vi "Send Initialize Parameters.vi"(7 "Message Priority (Normal)":T2=enum."Normal", 8 "error in (no error)":errorcluster, 10 "Cluster":T1={"Save Options"={"Primary Storage Location"=path "", "Backup Storage Location"=path "", "Enable Primary"=FALSE, "Enable Secondary"=FALSE, "Save Image as"=enum."RAW"}, "Other Settings"={"Show Image Averaging Option"=TRUE, "Component Name Prefix"=""}, "PLC Parameters"={"Initialize Parameters"={"VISA  Port"="", "Baud Rate"=0}, "Wakeup Bit (Set)"={"Address"=0, "Set/Reset"=FALSE}, "Incoming Bit (Get)"={"Address"=0, "Set/Reset"=FALSE}, "Acknowledge Bit (Set)"={"Address"=0, "Set/Reset"=FALSE}}}, 11 "Message Enqueuer":refnum<class "Message Enqueuer.lvclass">) -> (0 "error out":errorcluster, 3 "Message Enqueuer out":refnum<class "Message Enqueuer.lvclass">)   [LabVIEW 2022 SP3, in "Controller.lvlib" / "Initialize Parameters Msg.lvclass"]
doc: "This VI sends the message to an actor."
uses:
  Initialize Parameters Msg.lvclass
  <vilib>/ActorFramework/Message Enqueuer/Message Enqueuer.lvclass
  <vilib>/ActorFramework/Message Enqueuer/Message Priority.ctl
  C:/Program Files/National Instruments/LabVIEW 2022/vi.lib/ActorFramework/Message/Message.lvclass
  Initialize Parameters Msg.lvclass/Initialize Parameters Msg.ctl
  <vilib>/ActorFramework/Message Enqueuer/Message Enqueuer.lvclass/Message Enqueuer.ctl
  <vilib>/ActorFramework/Message Priority Queue/Priority Enqueue.vi
  E:/image-harvest/Controller/Controller Messages/Initialize Parameters Msg/Initialize Parameters Msg.lvclass
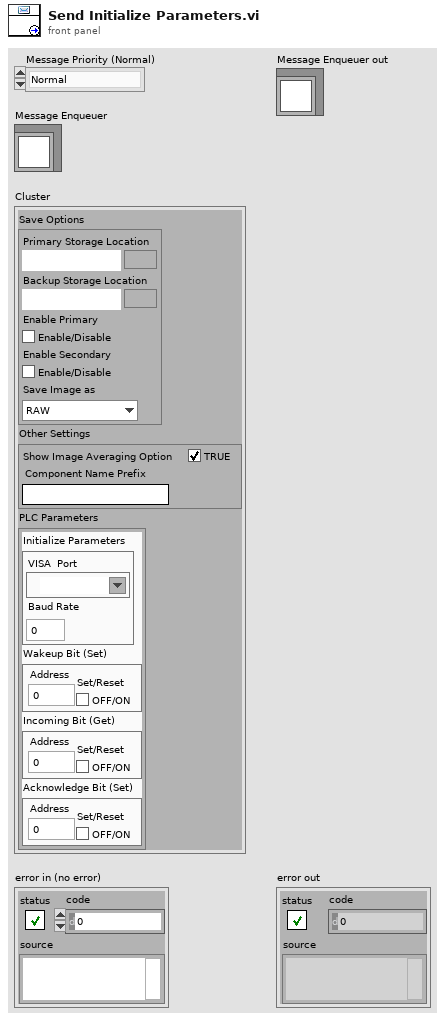
[diagram p1: front panel]
types:
  T1 = cluster{"Save Options":cluster{"Primary Storage Location":path, "Backup Storage Location":path, "Enable Primary":bool, "Enable Secondary":bool, "Save Image as":enum16{"RAW", "TIFF"}}, "Other Settings":cluster{"Show Image Averaging Option":bool, "Component Name Prefix":string}, "PLC Parameters":cluster{"Initialize Parameters":cluster{"VISA  Port":refnum<visa-resource-name>, "Baud Rate":u32}, "Wakeup Bit (Set)":cluster{"Address":u16, "Set/Reset":bool}, "Incoming Bit (Get)":cluster{"Address":u16, "Set/Reset":bool}, "Acknowledge Bit (Set)":cluster{"Address":u16, "Set/Reset":bool}}}
  T2 = typedef "Actor Framework.lvlib/Message Enqueuer.lvclass/Message Priority.ctl" = enum16{"Low", "Normal", "High"}
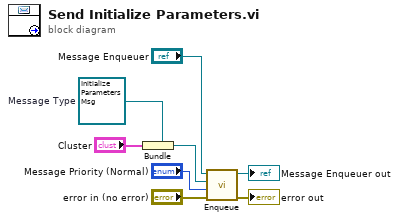
[diagram p0: block diagram]
diagram:
  w5 = refnum<class "Initialize Parameters Msg.lvclass"> refnum  # Message Type
  n1 = Bundle(cluster=w5, "Cluster") -> (w4:refnum<class "Initialize Parameters Msg.lvclass">)
  n2 = call <vilib>:"Enqueue.vi"("error in (no error)"="error in (no error)", "Message Priority (Normal)"="Message Priority (Normal)", "Message"=w4, "Message Enqueuer in"="Message Enqueuer") -> ("error out"=→"error out":errorcluster, "Message Enqueuer in"=→"Message Enqueuer out":refnum<class "Message Enqueuer.lvclass">)  [unwired: 6 in]
